vi "SV TDMS Read Speed Profile (1 Ch).vi"(0 "tdms file":refnum<k34>, 5 "group name in":string="SpeedProfile", 7 "channel name in":string="Channel0", 11 "error in":errorcluster) -> (3 "scale labels":T2, 4 "tdms file out":refnum<k34>, 6 "group name out":string, 8 "channel name out":string, 10 "speed profile":T3 {"speed [RPM]" format="%.2f"; "time [s]" format="%.2f"}, 13 "speed position info":T1, 15 "error out":errorcluster)   [LabVIEW 2017]
doc: "Reads the specified .tdms file and returns data in a format specific to the polymorphic instance selected."
uses:
  <vilib>/addons/_NISVFA/_Shared subVIs/Controls/svc_Speed Profile.ctl
  <vilib>/addons/_NISVFA/_Shared subVIs/Controls/svc_Position Info.ctl
  <vilib>/addons/_NISVFA/_Shared subVIs/Controls/NI Channel Properties.ctl
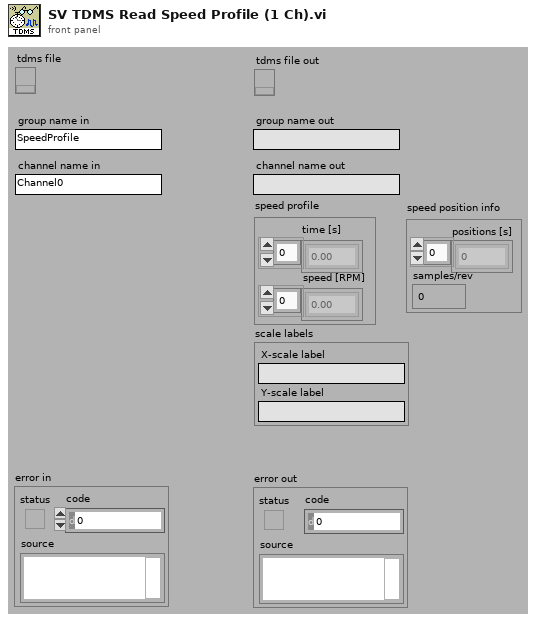
[diagram p1: front panel]
types:
  T1 = typedef "svc_Position Info.ctl" = cluster{"positions [s]":dbl[], "samples/rev":dbl}
  T2 = cluster{"X-scale label":string, "Y-scale label":string}
  T3 = typedef "svc_Speed Profile.ctl" = cluster{"time [s]":dbl[], "speed [RPM]":dbl[]}
  T4 = typedef "NI Channel Properties.ctl" = u16
  T5 = cluster{"scale label with units":string, "scale label with units":string}
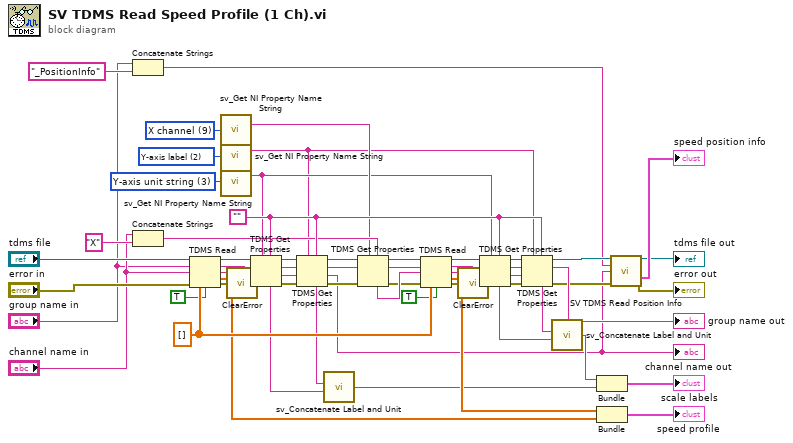
[diagram p0: block diagram]
diagram:
  w40 = T4 3 items=["Channel name", "Channel description", "Y-axis label", "Y-axis unit string", "X-axis label", "X-axis unit string", "x0", "dx", "Number of samples", "X channel", "Filter settled", "dB reference", "Window", "Window parameter", "Window size", "FFT size", "Peak units", "Spectrum type", "Magnitude scale", "Spectral density", "Sensor sensitivity (mV/EU)", "X-axis domain", "LabVIEW datatype"] ("property")
  w41 = T4 2 items=["Channel name", "Channel description", "Y-axis label", "Y-axis unit string", "X-axis label", "X-axis unit string", "x0", "dx", "Number of samples", "X channel", "Filter settled", "dB reference", "Window", "Window parameter", "Window size", "FFT size", "Peak units", "Spectrum type", "Magnitude scale", "Spectral density", "Sensor sensitivity (mV/EU)", "X-axis domain", "LabVIEW datatype"] ("property")
  w43 = T4 9 items=["Channel name", "Channel description", "Y-axis label", "Y-axis unit string", "X-axis label", "X-axis unit string", "x0", "dx", "Number of samples", "X channel", "Filter settled", "dB reference", "Window", "Window parameter", "Window size", "FFT size", "Peak units", "Spectrum type", "Magnitude scale", "Spectral density", "Sensor sensitivity (mV/EU)", "X-axis domain", "LabVIEW datatype"] ("property")
  w48 = "" ("X-axis label")
  w35 = dbl[] [] ("X")
  n1 = Concatenate Strings("group name in", "_PositionInfo") -> (w7:string)
  n2 = Concatenate Strings("channel name in", "X" ("string")) -> (w44:string)
  n3 = TDMS Read(0:"tdms file", 5:"group name in", 7:"channel name in", 11:"error in", 12:w35, 13:TRUE ("return channels in file order? (F)")) -> (4:w55:refnum<k34>, 6:w24:string, 8:w27:string, 10:w28:dbl[], 15:w3:errorcluster)  [unwired: 2 in, 1 out]
  n4 = call <vilib>:"sv_Get NI Property Name String.vi"("property"=w43) -> ("TDMS property name"=w42:string)  [unwired: 13 in, 1 out]
  n5 = call <vilib>:"sv_Get NI Property Name String.vi"("property"=w41) -> ("TDMS property name"=w38:string)  [unwired: 13 in, 1 out]
  n6 = call <vilib>:"sv_Get NI Property Name String.vi"("property"=w40) -> ("TDMS property name"=w39:string)  [unwired: 13 in, 1 out]
  n7 = call <vilib>:"ClearError.vi"("error in (no error)"=w3) -> ("error out"=w51:errorcluster)
  n8 = TDMS Get Properties(5:w48, 7:w39, 8:w51, 9:w27, 10:w24, 11:w55) -> (0:w50:errorcluster, 1:w54:string, 2:w53:string, 3:w49:refnum<k34>, 4:w15:string)  [unwired: 1 out]
  n9 = TDMS Get Properties(5:w48, 7:w38, 8:w50, 9:w54, 10:w53, 11:w49) -> (0:w47:errorcluster, 1:w6:string, 2:w46:string, 3:w45:refnum<k34>, 4:w16:string)  [unwired: 1 out]
  "channel name out" <- w6
  n10 = call <vilib>:"sv_Concatenate Label and Unit.vi"("unit string"=w15, "label"=w16) -> ("scale label with units"=w21:string)  [unwired: 4 in]
  n11 = TDMS Get Properties(5:w44, 7:w42, 8:w47, 10:w46, 11:w45) -> (0:w31:errorcluster, 2:w33:string, 3:w34:refnum<k34>, 4:w32:string)  [unwired: 1 in, 2 out]
  n12 = TDMS Read(0:w34, 5:w33, 7:w32, 11:w31, 12:w35, 13:TRUE ("return channels in file order? (F)")) -> (4:w58:refnum<k34>, 6:w25:string, 8:w26:string, 10:w29:dbl[], 15:w4:errorcluster)  [unwired: 2 in, 1 out]
  n13 = call <vilib>:"ClearError.vi"("error in (no error)"=w4) -> ("error out"=w59:errorcluster)
  n14 = TDMS Get Properties(5:w48, 7:w39, 8:w59, 9:w26, 10:w25, 11:w58) -> (0:w5:errorcluster, 1:w56:string, 2:w57:string, 4:w17:string)  [unwired: 2 out]
  n15 = TDMS Get Properties(5:w48, 7:w38, 8:w5, 9:w56, 10:w57, 11:w58) -> (0:w10:errorcluster, 2:→"group name out":string, 3:w12:refnum<k34>, 4:w18:string)  [unwired: 2 out]
  n16 = call <vilib>:"sv_Concatenate Label and Unit.vi"("unit string"=w17, "label"=w18) -> ("scale label with units"=w22:string)  [unwired: 4 in]
  n17 = Bundle("scale label with units"=w22, "scale label with units"=w21) -> (→"scale labels":T5)  [unwired: 1 in]
  n18 = Bundle("X"=w29, "X"=w28) -> (→"speed profile":cluster{"X":dbl[], "X":dbl[]})  [unwired: 1 in]
  n19 = call <vilib>:"SV TDMS Read Position Info.vi"("tdms file"=w12, "group name in"=w7, "channel name in"=w6, "error in"=w10) -> ("tdms file out"=→"tdms file out":refnum<k34>, "position info"=→"speed position info":T1, "error out"=→"error out":errorcluster)  [unwired: 7 in, 2 out]
